vi "Signal analysis with T,P.vi"() -> ()   [LabVIEW 2014]
uses:
  <vilib>/Utility/error.llb/DialogType.ctl
  <vilib>/Utility/file.llb/Write To Spreadsheet File (DBL).vi
  <instrlib>/Fluke 884X Series/Public/Data/Read (Multiple Points).vi
  <instrlib>/Fluke 884X Series/Fluke 884X Series.lvlib
panel:
  out "Temperature Frequency":dbl
  out "Temperature Amplitude":dbl
  out "Pressure Frequency":dbl
  out "Pressure Amplitude":dbl
  in  "Write":bool
  in  "mkv per degree(thermocouple type)":dbl
  out "T,C":dbl
  out "T,K":dbl
  in  "Tkomn, C":dbl
  in  "Timeout":i32=10000
  in  "Sample Count (10)":i32=10
  in  "Manual Range (1.0)":dbl=1.0
  in  "Auto Range (T:Enable)":bool=TRUE
  in  "Function (0: DC Voltage)":u16(ring) items=["DC Voltage", "AC Voltage", "2 - Wire Resistance", "4 - Wire Resistance", "DC Current", "AC Current", "Frequency", "Period", "Continuity", "Diode Checking", "Temperature", "Capacitance"]
  in  "Manual Resolution (5.5 Digits)":dbl(ring)=5.5 items=["4.5"=4.5, "5.5"=5.5, "6.5"=6.5]
  out "Temperature":dbl
  out "Temperature from Fluke884X":dbl[](graph)
  in  "Serial Configuration":T1={"Baud Rate"=9600, "Parity"=0, "Data Bits"=8, "Stop Bits"=10, "Flow Control"=0} {"Flow Control" items=["None", "XON/XOFF", "RTS/CTS", "XON/XOFF & RTS/CTS", "DTR/DSR", "XON/XOFF & DTR/DSR"]; "Stop Bits" items=["1.0"=10, "1.5"=15, "2.0"=20]; "Data Bits" items=["7"=7, "8"=8]; "Parity" items=["None", "Odd", "Even", "Mark", "Space"]; "Baud Rate" items=["300"=300, "600"=600, "1200"=1200, "2400"=2400, "4800"=4800, "9600"=9600, "19200"=19200]}
  in  "VISA resource name":refnum<visa-resource-name>
  in  "Write Raw  signal temperature":bool
  in  "Write Raw signal pressure":bool
  in  "stop":bool
  in  "Write Signal Statistics":bool
  out "Waveform Graph 3":dynamicdata(graph)
  out "Waveform Graph 2":dynamicdata(graph)
  in  "Filter 2":bool
  in  "Filter":bool
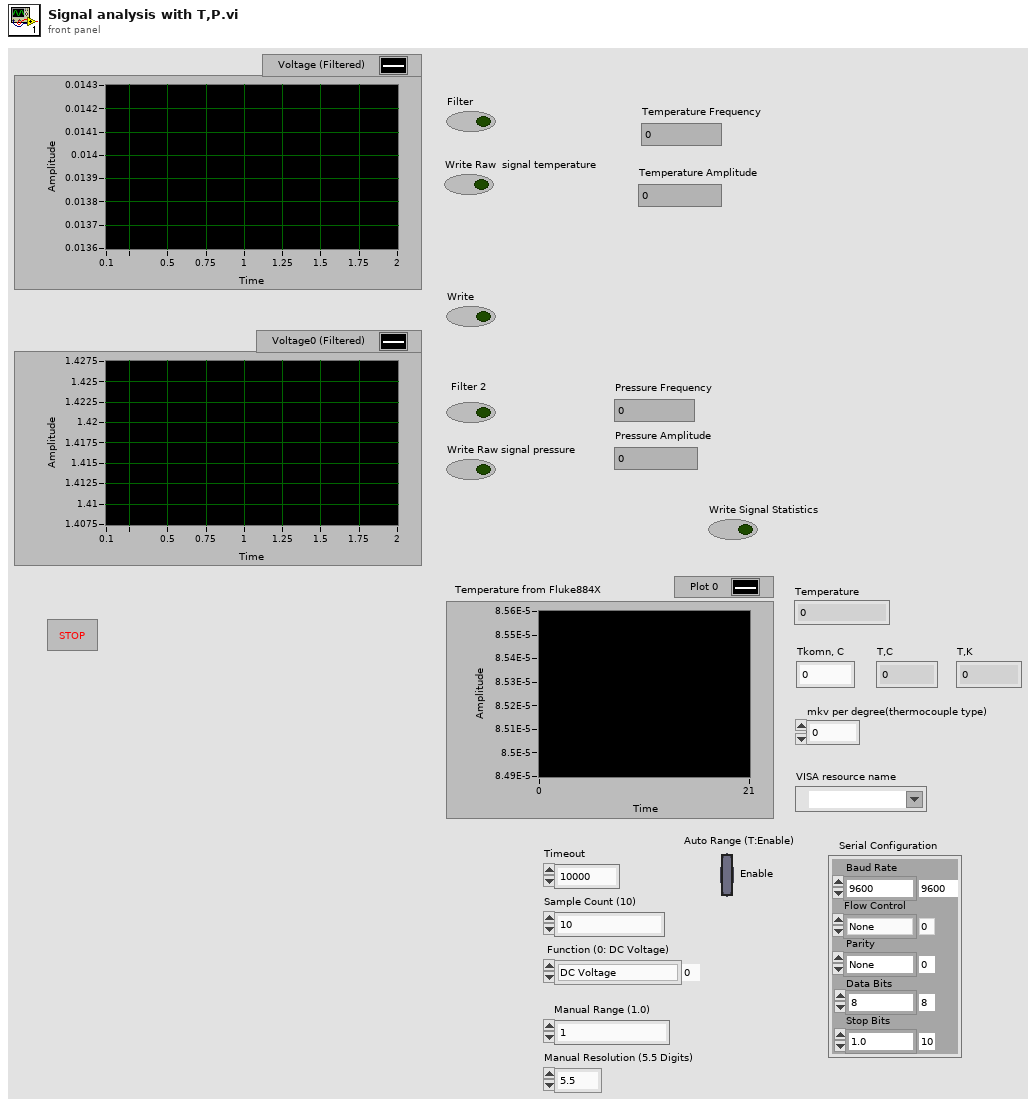
[diagram p1: front panel]
types:
  T1 = cluster{"Baud Rate":u32, "Parity":u16, "Data Bits":u16, "Stop Bits":u16, "Flow Control":u16}
  T2 = typedef "DialogType.ctl" = u16
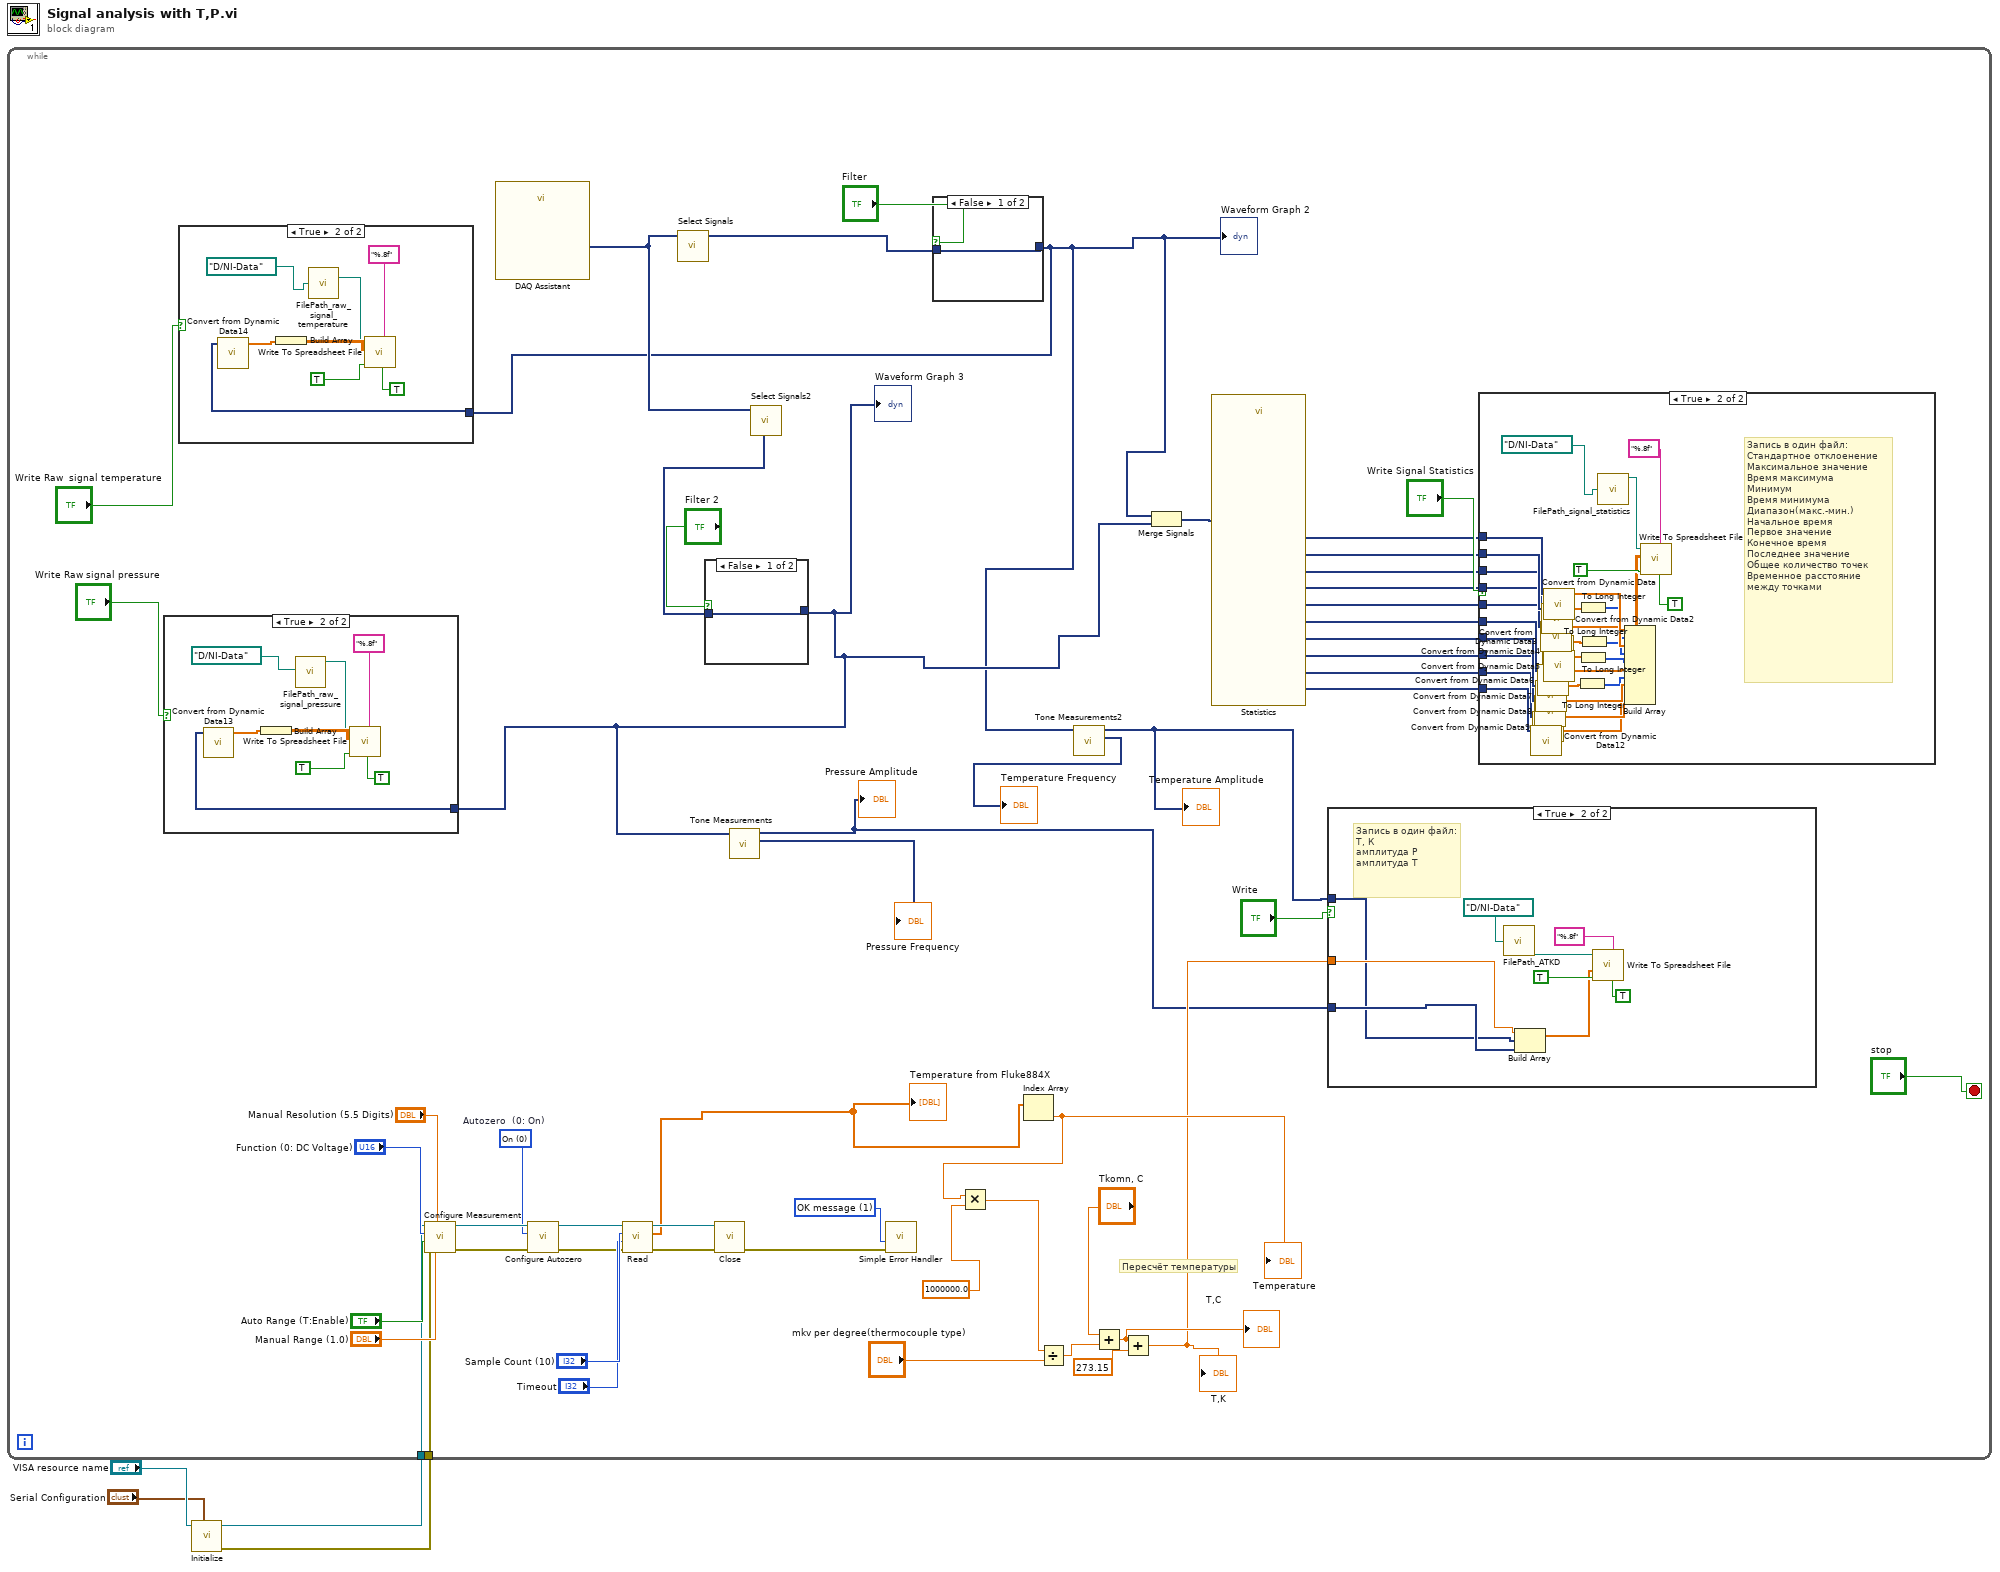
[diagram p0: block diagram]
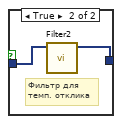
[diagram p6: hidden frame]
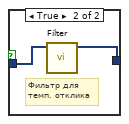
[diagram p7: hidden frame]
diagram:
  n1 = call <instrlib>:"Initialize.vi"("Serial Configuration"="Serial Configuration", "VISA resource name"="VISA resource name") -> ("error out"=w1:errorcluster, "VISA resource name out"=w2:refnum<visa-resource-name>)  [unwired: 8 in]
  n2 = while {
    tunnel: w2 -> [w14]
    tunnel: w1 -> [w13]
    stop <- "stop" stop-if-true
    w24 = u16 0 items=["On", "Off", "Once"]  # Autozero  (0: On)
    w38 = T2 1 items=["no dialog", "OK message", "continue or stop message", "OK message + warnings", "continue/stop + warnings"] ("type of dialog (OK msg:1)")
    # "Пересчёт температуры"
    n3 = call <instrlib>:"Configure Measurement.vi"("Manual Range (1.0)"="Manual Range (1.0)", "Manual Resolution (5.5 Digits)"="Manual Resolution (5.5 Digits)", "error in (no error)"=w13, "Auto Range (T:Enable)"="Auto Range (T:Enable)", "Function (0: DC Voltage)"="Function (0: DC Voltage)", "VISA resource name"=w14) -> ("error out"=w28:errorcluster, "VISA resource name out"=w27:refnum<visa-resource-name>)  [unwired: 4 in]
    n4 = call "DAQ Assistant"() -> ("data"=w40:dynamicdata)  [unwired: 2 in, 9 out]
    n5 = call <instrlib>:"Configure Autozero.vi"("error in (no error)"=w28, "Autozero  (0: On)"=w24, "VISA resource name"=w27) -> ("error out"=w25:errorcluster, "VISA resource name out"=w26:refnum<visa-resource-name>)  [unwired: 7 in]
    n6 = call-poly <instrlib>:"Read.vi"("error in (no error)"=w25, "Timeout (10000 ms)"="Timeout", "Sample Count (1)"="Sample Count (10)", "VISA resource name"=w26) -> ("error out"=w35:errorcluster, "Measurements"=w19:dbl[], "VISA resource name out"=w36:refnum<visa-resource-name>)  [unwired: 5 in]
    "Temperature from Fluke884X" <- w19
    n7 = call "Select Signals"("Signals"=w40) -> ("Signal Out"=w39:dynamicdata)  [unwired: 1 in, 9 out]
    n8 = call <instrlib>:"Close.vi"("error in (no error)"=w35, "VISA resource name"=w36) -> ("error out"=w37:errorcluster)  [unwired: 9 in]
    n9 = call "Select Signals2"("Signals"=w40) -> ("Signal Out"=w57:dynamicdata)  [unwired: 1 in, 9 out]
    n10 = case shown="False" "Filter 2" {
      tunnel: w57 -> [w114 w116]
      tunnel: [w114 w115] -> w9
      frame False {
      }
      frame True {
        # "Фильтр для\nтемп. отклика"
        n11 = call "Filter2"("Signal"=w116) -> ("Filtered Signal"=w115:dynamicdata)  [unwired: 2 in, 8 out]
      }
    }
    "Waveform Graph 3" <- w9
    n12 = case shown="True" "Write Raw signal pressure" {
      tunnel: w9 -> [_ w78]
      frame False {
      }
      frame True {
        n13 = call "Convert from Dynamic Data13"("Dynamic Data Type"=w78) -> ("Array"=w79:dbl[])  [unwired: 3 in]
        n14 = Build Array(w79) -> (w80:dbl[][])
        n15 = call "FilePath_raw_signal_pressure.vi"("base folder path"=path "D:/NI-Data") -> ("Raw_data_path"=w76:path)  [unwired: 3 in]
        n16 = call-poly <vilib>:"Write To Spreadsheet File.vi"("transpose? (no:F)"=TRUE, "format (%.3f)"="%.8f", "append to file? (new file:F)"=TRUE, "2D data"=w80, "file path (dialog if empty)"=w76) -> ()  [unwired: 1 in, 3 out]
      }
    }
    n17 = call "Tone Measurements"("Signals"=w9) -> ("Frequency"=→"Pressure Frequency":dynamicdata, "Amplitude"=w8:dynamicdata)  [unwired: 1 in, 8 out]
    "Pressure Amplitude" <- w8
    n18 = call <vilib>:"Simple Error Handler.vi"("type of dialog (OK msg:1)"=w38, "error in (no error)"=w37) -> ()  [unwired: 3 in, 5 out]
    n19 = case shown="False" "Filter" {
      tunnel: w39 -> [w117 w119]
      tunnel: [w117 w118] -> w7
      frame False {
      }
      frame True {
        # "Фильтр для\nтемп. отклика"
        n20 = call "Filter"("Signal"=w119) -> ("Filtered Signal"=w118:dynamicdata)  [unwired: 2 in, 8 out]
      }
    }
    "Waveform Graph 2" <- w7
    n21 = case shown="True" "Write Raw  signal temperature" {
      tunnel: w7 -> [_ w70]
      frame False {
      }
      frame True {
        n22 = call "Convert from Dynamic Data14"("Dynamic Data Type"=w70) -> ("Array"=w71:dbl[])  [unwired: 3 in]
        n23 = Build Array(w71) -> (w72:dbl[][])
        n24 = call "FilePath_raw_signal_temperature.vi"("base folder path"=path "D:/NI-Data") -> ("Raw_data_path"=w69:path)  [unwired: 3 in]
        n25 = call-poly <vilib>:"Write To Spreadsheet File.vi"("transpose? (no:F)"=TRUE, "format (%.3f)"="%.8f", "append to file? (new file:F)"=TRUE, "2D data"=w72, "file path (dialog if empty)"=w69) -> ()  [unwired: 1 in, 3 out]
      }
    }
    n26 = Index Array(array=w19) -> (element=w17:dbl)  [unwired: 1 in]
    "Temperature" <- w17
    n27 = Multiply(x=w17, y=1000000.0) -> (x*y=w15:dbl)
    n28 = Divide(x=w15, y="mkv per degree(thermocouple type)") -> (x/y=w22:dbl)
    n29 = call "Tone Measurements2"("Signals"=w7) -> ("Frequency"=→"Temperature Frequency":dynamicdata, "Amplitude"=w6:dynamicdata)  [unwired: 1 in, 8 out]
    "Temperature Amplitude" <- w6
    n30 = Add(x="Tkomn, C", y=w22) -> (x+y=w20:dbl)
    "T,C" <- w20
    n31 = Add(x=w20, y=273.15) -> (x+y=w12:dbl)
    "T,K" <- w12
    n32 = Merge Signals(w7, w9) -> (w43:dynamicdata)
    n33 = call "Statistics"("Signals"=w43) -> ("Total Samples"=w45:dynamicdata, "Time Delta"=w44:dynamicdata, "Last Value"=w46:dynamicdata, "Last Time"=w47:dynamicdata, "First Value"=w48:dynamicdata, "First Time"=w49:dynamicdata, "Time of Minimum"=w50:dynamicdata, "Minimum"=w51:dynamicdata, "Time of Maximum"=w52:dynamicdata, "Maximum"=w53:dynamicdata)  [unwired: 16 in, 1 out]
    n34 = case shown="True" "Write" {
      tunnel: w12 -> [_ w61]
      tunnel: w8 -> [_ w60]
      tunnel: w6 -> [_ w59]
      frame False {
      }
      frame True {
        # "Запись в один файл:\nТ, К\nамплитуда P\nамплитуда Т"
        n35 = call "FilePath_ATKD.vi"("base folder path"=path "D:/NI-Data") -> ("ATKD"=w67:path)  [unwired: 3 out]
        n36 = Build Array(w61, w59, w60) -> (w62:dbl[])
        n37 = call-poly <vilib>:"Write To Spreadsheet File.vi"("transpose? (no:F)"=TRUE, "format (%.3f)"="%.8f", "append to file? (new file:F)"=TRUE, "1D data"=w62, "file path (dialog if empty)"=w67) -> ()  [unwired: 1 in, 3 out]
      }
    }
    n38 = case shown="True" "Write Signal Statistics" {
      tunnel: w53 -> [_ w107]
      tunnel: w52 -> [_ w106]
      tunnel: w51 -> [_ w105]
      tunnel: w50 -> [_ w104]
      tunnel: w49 -> [_ w103]
      tunnel: w48 -> [_ w102]
      tunnel: w47 -> [_ w101]
      tunnel: w46 -> [_ w100]
      tunnel: w45 -> [_ w99]
      tunnel: w44 -> [_ w98]
      frame False {
      }
      frame True {
        # "Запись в один файл:\nСтандартное отклоенение\nМаксимальное значение\nВремя максимума\nМинимум\nВремя минимума\nДиапазон(макс.-мин.)\nНачальное время\nПервое значение\nКонечное время\nПоследнее значение\nОбщее количество точек\nВременное расстояние между точками"
        n39 = call "Convert from Dynamic Data12"("Dynamic Data Type"=w98) -> ("Array"=w93:dbl[])  [unwired: 3 in]
        n40 = call "Convert from Dynamic Data9"("Dynamic Data Type"=w99) -> ("Array"=w94:dbl[])  [unwired: 3 in]
        n41 = call "Convert from Dynamic Data8"("Dynamic Data Type"=w100) -> ("Array"=w95:dbl[])  [unwired: 3 in]
        n42 = call "Convert from Dynamic Data7"("Dynamic Data Type"=w101) -> ("Array"=w85:dbl[])  [unwired: 3 in]
        n43 = call "Convert from Dynamic Data6"("Dynamic Data Type"=w102) -> ("Array"=w86:dbl[])  [unwired: 3 in]
        n44 = call "Convert from Dynamic Data3"("Dynamic Data Type"=w105) -> ("Array"=w96:dbl[])  [unwired: 3 in]
        n45 = call "Convert from Dynamic Data2"("Dynamic Data Type"=w106) -> ("Array"=w90:dbl[])  [unwired: 3 in]
        n46 = call "Convert from Dynamic Data4"("Dynamic Data Type"=w104) -> ("Array"=w92:dbl[])  [unwired: 3 in]
        n47 = call "Convert from Dynamic Data"("Dynamic Data Type"=w107) -> ("Array"=w97:dbl[])  [unwired: 3 in]
        n48 = call "Convert from Dynamic Data5"("Dynamic Data Type"=w103) -> ("Array"=w88:dbl[])  [unwired: 3 in]
        n49 = To Long Integer(number=w85) -> (32bit integer=w84:i32[])
        n50 = To Long Integer(number=w90) -> (32bit integer=w89:i32[])
        n51 = To Long Integer(number=w88) -> (32bit integer=w87:i32[])
        n52 = To Long Integer(number=w92) -> (32bit integer=w91:i32[])
        n53 = call "FilePath_signal_statistics.vi"("base folder path"=path "D:/NI-Data") -> ("Signal_path"=w108:path)  [unwired: 3 in]
        n54 = Build Array(w97, w89, w96, w91, w87, w86, w84, w95, w94, w93) -> (w110:dbl[][])
        n55 = call-poly <vilib>:"Write To Spreadsheet File.vi"("transpose? (no:F)"=TRUE, "format (%.3f)"="%.8f", "append to file? (new file:F)"=TRUE, "2D data"=w110, "file path (dialog if empty)"=w108) -> ()  [unwired: 1 in, 3 out]
      }
    }
  }
